vi "ts_tree_set_glyphs.vi"(8 "error in":errorcluster, 11 "Tree.in":refnum<vi>) -> (0 "error out":errorcluster, 3 "Tree.out":refnum<vi>)   [LabVIEW 2015]
doc: "sets the custom item symbols used by this application - perform during initialization"
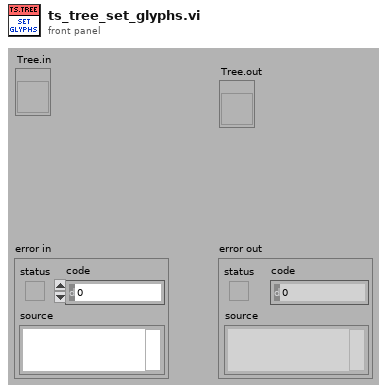
[diagram p1: front panel]
types:
  T1 = typedef "imagedata.ctl" = cluster{"image type":i32, "image depth":i32, "image":u8[], "mask":u8[], "colors":u32[], "Rectangle":cluster{"left":i16, "top":i16, "right":i16, "bottom":i16}}
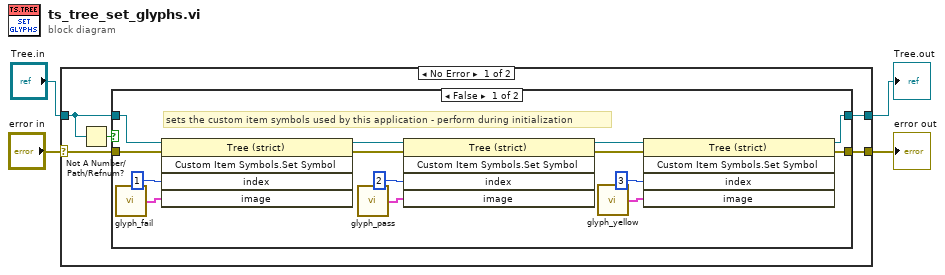
[diagram p0: block diagram]
diagram:
  n1 = case shown="No Error" "error in" {
    selector: "error in" -> [w9 w26]
    tunnel: "Tree.in" -> [w5 w27]
    tunnel: [w7 w27] -> w2
    tunnel: [w8 w26] -> w1
    frame No Error {
      n2 = Not A Number/Path/Refnum?(number/path/refnum=w5) -> (NaN/Path/Refnum?=w6:bool)
      n3 = case shown="False" w6 {
        tunnel: w5 -> [w21 w25]
        tunnel: w9 -> [w16 w24]
        tunnel: [w13 w24] -> w8
        tunnel: [w12 w25] -> w7
        frame False {
          # "sets the custom item symbols used by this application - perform during initialization"
          n4 = call "glyph_fail.vi"() -> ("image data"=w18:T1)  [unwired: 5 in]
          n5 = invoke class="Tree (strict)" method="Custom Item Symbols.Set Symbol"(reference=w21, error in=w16, "index"=1 ("Index"), "image"=w18) -> (reference out=w20:refnum<vi>, error out=w19:errorcluster)  [unwired: 1 in, 3 out]
          n6 = call "glyph_pass.vi"() -> ("image data"=w23:T1)  [unwired: 5 in]
          n7 = invoke class="Tree (strict)" method="Custom Item Symbols.Set Symbol"(reference=w20, error in=w19, "index"=2 ("Index"), "image"=w23) -> (reference out=w15:refnum<vi>, error out=w14:errorcluster)  [unwired: 1 in, 3 out]
          n8 = call "glyph_yellow.vi"() -> ("image data"=w10:T1)  [unwired: 5 in]
          n9 = invoke class="Tree (strict)" method="Custom Item Symbols.Set Symbol"(reference=w15, error in=w14, "index"=3 ("Index"), "image"=w10) -> (reference out=w12:refnum<vi>, error out=w13:errorcluster)  [unwired: 1 in, 3 out]
        }
        frame True {
        }
      }
    }
    frame Error {
    }
  }
  "Tree.out" <- w2
  "error out" <- w1
